vi "ParaCompare.vi"(8 "error in (no error)":errorcluster caption="错误输入（无错误）", 10 "参数输出":T2={"帧ID1"=1617, "等待延时"=10, "间隔延时"=0, "总时间"=1, "总次数"=2, "发送数据1"="1122334455667788", "接收数据1"="1122334455667788", "发送数据2"="1122334455667788", "接收数据2"="1122334455667788", "CAN盒类型"=3, "帧ID2"=1539, "同步启动个数"=8, "模式"=enum."单个", "Baud"=12} {"Baud" items=["250k bps"=10, "10k bps"=2, "5k bps"=1, "50k bps"=5, "40k bps"=4, "20k bps"=3, "80k bps"=6, "100k bps"=7, "125k bps"=8, "200k bps"=9, "400k bps"=11, "500k bps"=12, "666k bps"=13, "800k bps"=14, "1000k bps"=15]; "帧ID2" format="%.0x"; "CAN盒类型" items=["PCI-CAN200"=7, "USB-CAN"=2, "USB-CAN200"=3]; "帧ID1" format="%.0x"}, 11 "原始参数":T2={"帧ID1"=1617, "等待延时"=10, "间隔延时"=0, "总时间"=1, "总次数"=2, "发送数据1"="1122334455667788", "接收数据1"="1122334455667788", "发送数据2"="1122334455667788", "接收数据2"="1122334455667788", "CAN盒类型"=3, "帧ID2"=1539, "同步启动个数"=3, "模式"=enum."单个", "Baud"=12} {"CAN盒类型" items=["PCI-CAN200"=7, "USB-CAN"=2, "USB-CAN200"=3]}) -> (0 "error out":errorcluster caption="错误输出", 3 "StrOut":string)   [LabVIEW 2013]
uses:
  USBCAN/DevType.ctl
panel:
  # "ms"
  # "ms"
  # "s"
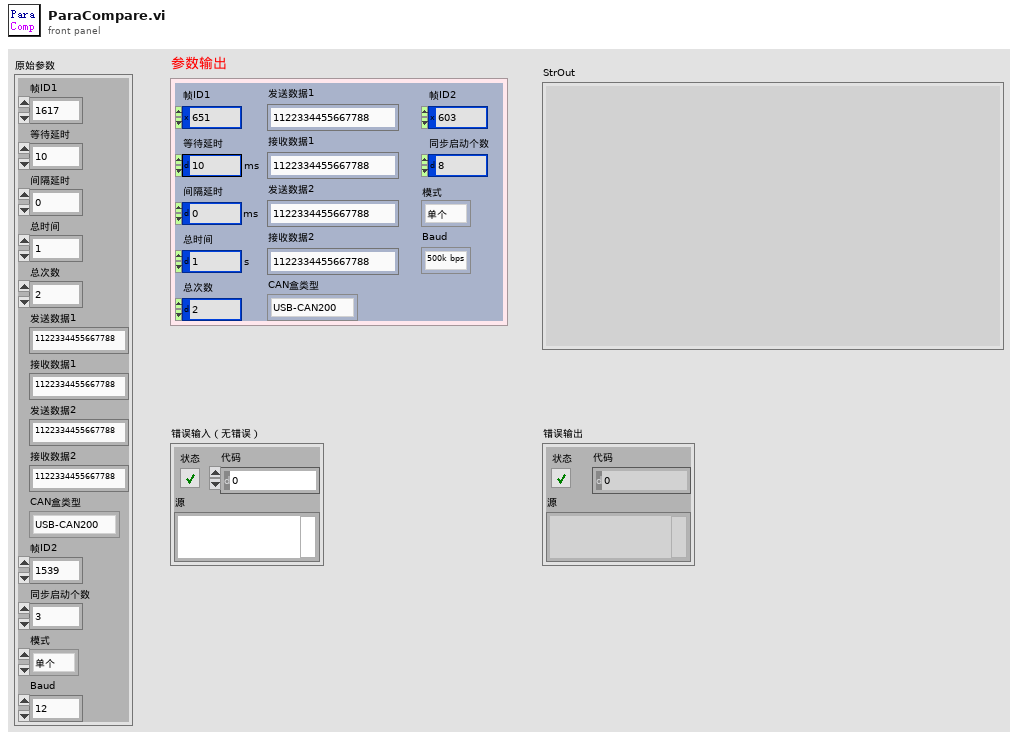
[diagram p1: front panel]
types:
  T1 = typedef "DevType.ctl" = u16
  T2 = cluster{"帧ID1":u32, "等待延时":u32, "间隔延时":u32, "总时间":u32, "总次数":u32, "发送数据1":string, "接收数据1":string, "发送数据2":string, "接收数据2":string, "CAN盒类型":T1, "帧ID2":u32, "同步启动个数":u8, "模式":enum16{"整体", "单个"}, "Baud":u8}
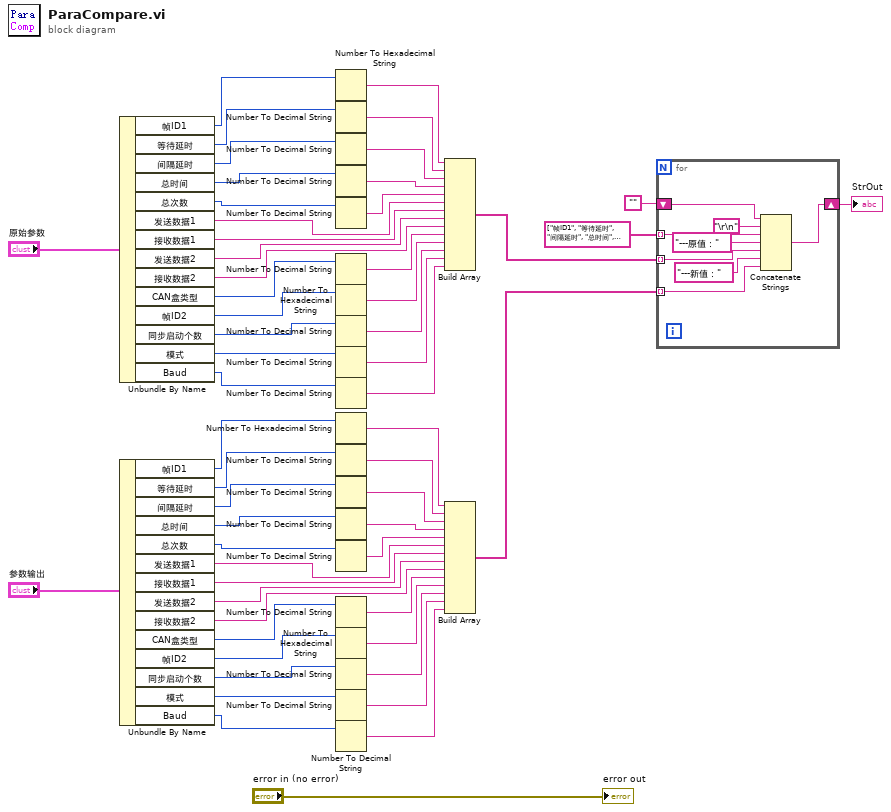
[diagram p0: block diagram]
diagram:
  n1 = Unbundle By Name("原始参数") -> ("帧ID1"=w55:u32, "等待延时"=w54:u32, "间隔延时"=w53:u32, "总时间"=w52:u32, "总次数"=w51:u32, "发送数据1"=w45:string, "接收数据1"=w44:string, "发送数据2"=w43:string, "接收数据2"=w42:string, "CAN盒类型"=w41:T1, "帧ID2"=w39:u32, "同步启动个数"=w37:u8, "模式"=w35:enum16{"整体", "单个"}, "Baud"=w33:u8)
  n2 = Unbundle By Name("参数输出") -> ("帧ID1"=w8:u32, "等待延时"=w9:u32, "间隔延时"=w10:u32, "总时间"=w11:u32, "总次数"=w12:u32, "发送数据1"=w18:string, "接收数据1"=w19:string, "发送数据2"=w20:string, "接收数据2"=w21:string, "CAN盒类型"=w22:T1, "帧ID2"=w24:u32, "同步启动个数"=w26:u8, "模式"=w28:enum16{"整体", "单个"}, "Baud"=w30:u8)
  n3 = Number To Hexadecimal String(2:w55) -> (0:w50:string)  [unwired: 1 in]
  n4 = Number To Decimal String(number=w54) -> (decimal integer string=w49:string)  [unwired: 1 in]
  n5 = Number To Decimal String(number=w53) -> (decimal integer string=w48:string)  [unwired: 1 in]
  n6 = Number To Decimal String(number=w52) -> (decimal integer string=w47:string)  [unwired: 1 in]
  n7 = Number To Decimal String(number=w51) -> (decimal integer string=w46:string)  [unwired: 1 in]
  n8 = Number To Decimal String(number=w41) -> (decimal integer string=w40:string)  [unwired: 1 in]
  n9 = Number To Hexadecimal String(2:w39) -> (0:w38:string)  [unwired: 1 in]
  n10 = Number To Decimal String(number=w37) -> (decimal integer string=w36:string)  [unwired: 1 in]
  n11 = Number To Decimal String(number=w35) -> (decimal integer string=w34:string)  [unwired: 1 in]
  n12 = Number To Decimal String(number=w33) -> (decimal integer string=w32:string)  [unwired: 1 in]
  n13 = Number To Hexadecimal String(2:w8) -> (0:w13:string)  [unwired: 1 in]
  n14 = Number To Decimal String(number=w9) -> (decimal integer string=w14:string)  [unwired: 1 in]
  n15 = Number To Decimal String(number=w10) -> (decimal integer string=w15:string)  [unwired: 1 in]
  n16 = Number To Decimal String(number=w11) -> (decimal integer string=w16:string)  [unwired: 1 in]
  n17 = Number To Decimal String(number=w12) -> (decimal integer string=w17:string)  [unwired: 1 in]
  n18 = Number To Decimal String(number=w22) -> (decimal integer string=w23:string)  [unwired: 1 in]
  n19 = Number To Hexadecimal String(2:w24) -> (0:w25:string)  [unwired: 1 in]
  n20 = Number To Decimal String(number=w26) -> (decimal integer string=w27:string)  [unwired: 1 in]
  n21 = Number To Decimal String(number=w28) -> (decimal integer string=w29:string)  [unwired: 1 in]
  n22 = Number To Decimal String(number=w30) -> (decimal integer string=w31:string)  [unwired: 1 in]
  n23 = Build Array(w50, w49, w48, w47, w46, w45, w44, w43, w42, w40, w38, w36, w34, w32) -> (w4:string[])
  n24 = Build Array(w13, w14, w15, w16, w17, w18, w19, w20, w21, w23, w25, w27, w29, w31) -> (w3:string[])
  n25 = for {
    shift-right: [w58] -> w2
    shift-left: "" -> [w57]
    tunnel: string[] ["帧ID1", "等待延时", "间隔延时", "总时间", "总次数", "发送数据1", "接收数据1", "发送数据2", "接收数据2", "CAN盒类型", "帧ID2", "同步启动个数", "模式", "Baud"] -> [w64] mode=indexing
    tunnel: w4 -> [w62] mode=indexing
    tunnel: w3 -> [w60] mode=indexing
    n26 = Concatenate Strings(w57, "\r\n", w64, "---原值：", w62, "---新值：", w60) -> (w58:string)
  }
  "StrOut" <- w2
  "error out" <- "error in (no error)"
